vi "Eagle_RT Create Pattern.vi"(0 "FPGA Reference":T3, 1 "Radius A":fxp<+/-,10,10>=180.0, 2 "Radius B":fxp<+/-,10,10>=180.0, 3 "Center":T4={"CX"=400.0, "CY"=300.0}, 5 "error in":errorcluster, 6 "One Shot":bool, 7 "Calib Values":T2={"X MULT"=0.0050048828125, "Y MULT"=0.0050048828125, "X OFFS"=-1.5, "Y OFFS"=-2.0}, 9 "Voltage Offset":T1={"VX OFFS"=-1.5, "VY OFFS"=-1.5}) -> (14 "FPGA Reference":T3, 19 "error out":errorcluster)   [LabVIEW 2015]
uses:
  Eagle RT FPGA Ref.ctl
  <vilib>/Utility/error.llb/Error Cluster From Error Code.vi
  <vilib>/rvi/errors/niLvFpgaAdjustHostInterfaceError.vi
  <vilib>/rvi/interface/nirviReadWriteControl/nirviReadWriteControl.xnode
  NiFpgaLv.dll
  <vilib>/rvi/interface/Simulation/niFpgaSimulationCallBeginRW.vi
  IP Dev Area/IP results.ctl
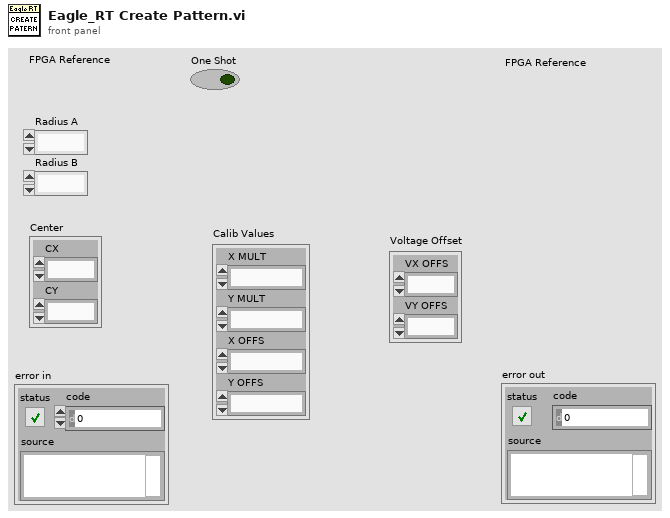
[diagram p1: front panel]
types:
  T1 = cluster{"VX OFFS":fxp<+/-,20,5>, "VY OFFS":fxp<+/-,20,5>}
  T2 = cluster{"X MULT":fxp<+/-,20,5>, "Y MULT":fxp<+/-,20,5>, "X OFFS":fxp<+/-,20,5>, "Y OFFS":fxp<+/-,20,5>}
  T3 = typedef "Eagle RT FPGA Ref.ctl" = refnum<k20>
  T4 = cluster{"CX":fxp<+/-,10,10>, "CY":fxp<+/-,10,10>}
  T5 = cluster{"PxMin":fxp<+,10,10>, "PxMax":fxp<+,10,10>, "PyMin":fxp<+,10,10>, "PyMax":fxp<+,10,10>}
  T6 = typedef "IP results.ctl" = cluster{"X":u16, "Y":u16, "A":dbl, "B":dbl, "Grade":u16, "Frame#":u16}
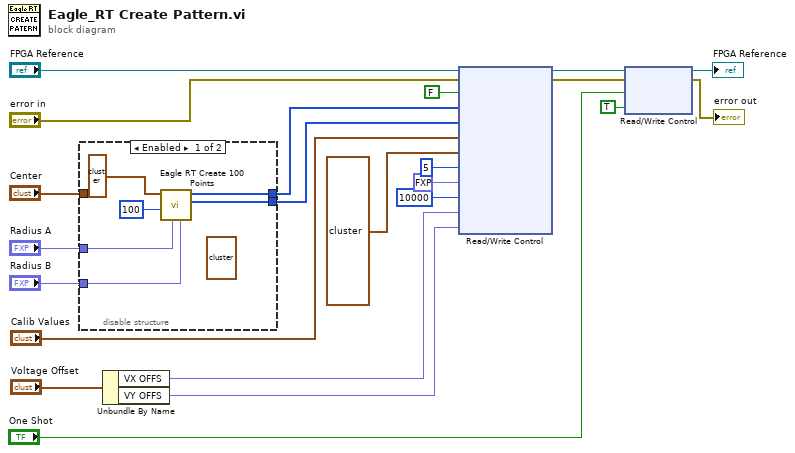
[diagram p0: block diagram]
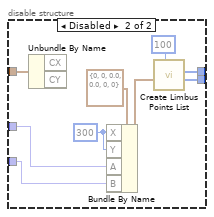
[diagram p2: hidden frame]
diagram:
  n1 = disable-structure shown="Enabled" {
    disable-tunnel: "Center" -> [_ w32]
    disable-tunnel: "Radius A" -> [w28 w31]
    disable-tunnel: "Radius B" -> [w27 w30]
    disable-tunnel: [w26 w35] -> w12
    disable-tunnel: [w25 w34] -> w11
    frame Enabled {
      (unwired) T4 {"CX"=300.0, "CY"=300.0} ("Center")
      n2 = call "Eagle RT Create 100 Points.vi"("Radius B"=w27, "Radius A"=w28, "NumOfPoints"=100, "Center"=T4 {"CX"=0.0, "CY"=0.0}) -> ("PY"=w25:i16[], "PX"=w26:i16[])  [unwired: 6 in]
    }
    frame Disabled {
      w29 = u16 300 ("X")
      n3 = Unbundle By Name(w32) -> ()  [unwired: 2 out]
      n4 = Bundle By Name(cluster=T6 {"X"=0, "Y"=0, "A"=0.0, "B"=0.0, "Grade"=0, "Frame#"=0} ("IP Results"), "X"=w29, "Y"=w29, "A"=w31, "B"=w30) -> (w36:T6)
      n5 = call "Create Limbus Points List.vi"("NoOfPoints"=u16 100, "IP Results"=w36) -> ("Y Points"=w34:i16[], "X Points"=w35:i16[])  [unwired: 8 in]
    }
  }
  n6 = Unbundle By Name("Voltage Offset") -> ("VX OFFS"=w5:fxp<+/-,20,5>, "VY OFFS"=w4:fxp<+/-,20,5>)
  n7 = xnode "Read/Write Control"("FPGA VI Reference In"="FPGA Reference", "error in"="error in", "Manual"=FALSE, "X Array"=w12, "Y Array"=w11, "Calib Values"="Calib Values", "NoGO Zone"=T5 {"PxMin"=400.0, "PxMax"=400.0, "PyMin"=300.0, "PyMax"=300.0}, "NumOfRetries"=u16 5, "Aim Ctrl"=fxp<+,16,3> 0.0, "ScanRate"=u32 10000, "VX OFFS"=w5, "VY OFFS"=w4) -> ("FPGA VI Reference Out"=w17:T3, "error out"=w16:errorcluster)
  n8 = xnode "Read/Write Control"("FPGA VI Reference In"=w17, "error in"=w16, "One Shot"="One Shot", "Enable"=TRUE) -> ("FPGA VI Reference Out"=→"FPGA Reference":T3, "error out"=→"error out":errorcluster)
